vi "Igor_Y_ITX.vi"(0 "concluding commnads":string="X preferences 1\nX KillStrings S_waveNames", 1 "starting commands":string="X preferences 0", 2 "window name":string="testwindow", 3 "Array":cluster{i32, dbl, "Power Spectrum":dbl[]}[](array[cluster]) {"Power Spectrum" format="%.2f"; "?" format="%.2f"}, 4 "y-column name":string="FFT", 5 "column extension":string[](array[string])=["0_01", "3_01", "6_01"], 6 "file":path=path "D:/work/data/BDATTP/ADA2") -> ()   [LabVIEW 2019]
uses:
  <vilib>/Utility/file.llb/Write To Spreadsheet File (DBL).vi
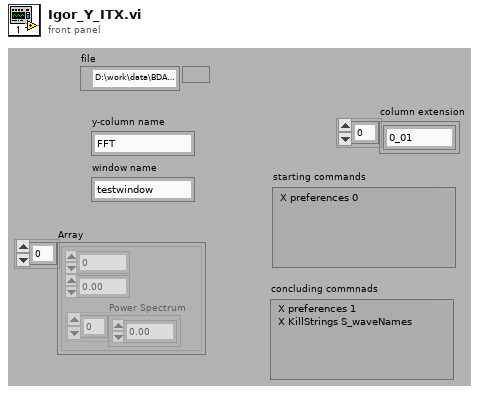
[diagram p1: front panel]
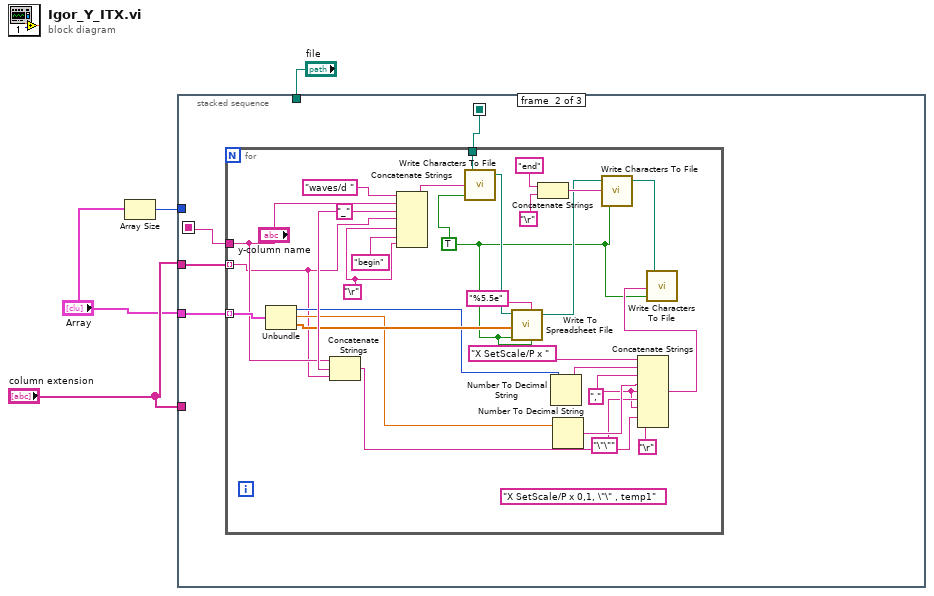
[diagram p0: block diagram]
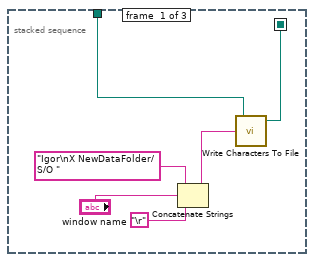
[diagram p2: hidden frame]
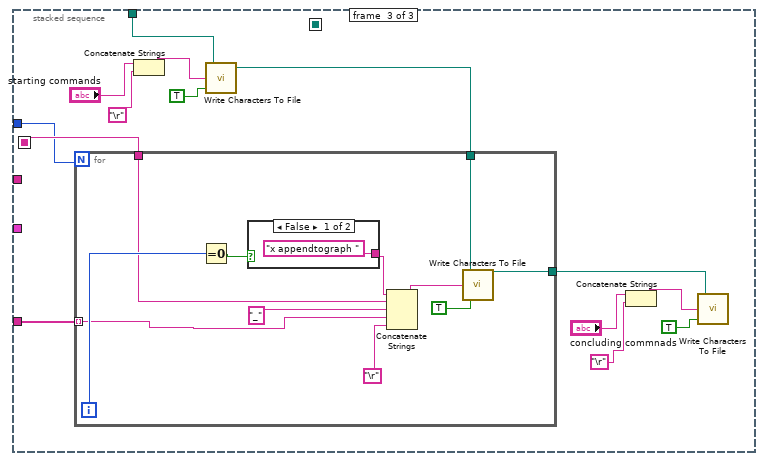
[diagram p3: hidden frame]
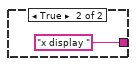
[diagram p4: hidden frame]
diagram:
  n1 = Array Size(array="Array") -> (size(s)=w3:i32)
  n2 = stacked-sequence {
    seq-local: [_ w12 _] -> [_ _ w45]
    seq-local: [w5 _ _] -> [_ w11 _]
    tunnel: "file" -> [w6 _ w46]
    tunnel: "column extension" -> [_ w14 _]
    tunnel: "Array" -> [_ w13 _]
    tunnel: "column extension" -> [_ _ w44]
    tunnel: w3 -> [_ _ w43]
    frame #0 {
      n3 = Concatenate Strings("Igor\nX NewDataFolder/S/O " ("character string"), "window name", "\r") -> (w8:string)
      n4 = call <vilib>:"Write Characters To File.vi"("character string"=w8, "file path (dialog if empty)"=w6) -> ("new file path (Not A Path if cancelled)"=w5:path)  [unwired: 3 in]
    }
    frame #1 {
      n5 = for {
        tunnel: w11 -> [w37]
        tunnel: w14 -> [w20] mode=indexing
        tunnel: w13 -> [w36] mode=indexing
        tunnel: ["y-column name"] -> w12
        (unwired) "X SetScale/P x 0,1, \"\" , temp1"
        w22 = ","
        w38 = "\r"
        w39 = "_"
        w15 = TRUE ("append to file? (new file:F)")
        n6 = Unbundle(w36) -> (w28:i32, w27:dbl, "Power Spectrum"=w29:dbl[])
        n7 = Concatenate Strings("y-column name", w39, w20) -> (w19:string)
        n8 = Concatenate Strings("waves/d ", "y-column name", w39, w20, w38, "begin", w38) -> (w40:string)
        n9 = call <vilib>:"Write Characters To File.vi"("append to file? (new file:F)"=w15, "character string"=w40, "file path (dialog if empty)"=w37) -> ("new file path (Not A Path if cancelled)"=w34:path)  [unwired: 2 in]
        n10 = call-poly <vilib>:"Write To Spreadsheet File.vi"("transpose? (no:F)"=w15, "format (%.3f)"="%5.5e", "append to file? (new file:F)"=w15, "1D data"=w29, "file path (dialog if empty)"=w34) -> ("new file path (Not A Path if cancelled)"=w30:path)  [unwired: 3 in]
        n11 = Concatenate Strings("end", "\r") -> (w31:string)
        n12 = Number To Decimal String(number=w28) -> (decimal integer string=w25:string)  [unwired: 1 in]
        n13 = Number To Decimal String(number=w27) -> (decimal integer string=w24:string)  [unwired: 1 in]
        n14 = call <vilib>:"Write Characters To File.vi"("append to file? (new file:F)"=w15, "character string"=w31, "file path (dialog if empty)"=w30) -> ("new file path (Not A Path if cancelled)"=w16:path)  [unwired: 2 in]
        n15 = Concatenate Strings("X SetScale/P x ", w25, w22, w24, w22, "\"\"", w22, w19, "\r") -> (w17:string)
        n16 = call <vilib>:"Write Characters To File.vi"("append to file? (new file:F)"=w15, "character string"=w17, "file path (dialog if empty)"=w16) -> ()  [unwired: 2 in, 1 out]
      }
    }
    frame #2 {
      n17 = Concatenate Strings("starting commands", "\r") -> (w54:string)
      n18 = call <vilib>:"Write Characters To File.vi"("append to file? (new file:F)"=TRUE, "character string"=w54, "file path (dialog if empty)"=w46) -> ("new file path (Not A Path if cancelled)"=w53:path)  [unwired: 2 in]
      n19 = for {
        N: w43 -> [_]
        tunnel: w53 -> [w67]
        tunnel: [w66] -> w49
        tunnel: w45 -> [w60]
        tunnel: w44 -> [w59] mode=indexing
        i -> [w62]
        n20 = Equal To 0?(x=w62) -> (x = 0?=w61:bool)
        n21 = case shown="False" w61 {
          tunnel: ["x appendtograph " "x display "] -> w63
          frame False {
          }
          frame True {
          }
        }
        n22 = Concatenate Strings(w63, w60, "_", w59, "\r") -> (w65:string)
        n23 = call <vilib>:"Write Characters To File.vi"("append to file? (new file:F)"=TRUE, "character string"=w65, "file path (dialog if empty)"=w67) -> ("new file path (Not A Path if cancelled)"=w66:path)  [unwired: 2 in]
      }
      n24 = Concatenate Strings("concluding commnads", "\r") -> (w50:string)
      n25 = call <vilib>:"Write Characters To File.vi"("append to file? (new file:F)"=TRUE, "character string"=w50, "file path (dialog if empty)"=w49) -> ()  [unwired: 2 in, 1 out]
    }
  }
